vi "myPID.vi"(11 "Numeric":dbl format="%#_13g") -> (3 "Numeric 2":dbl)   [LabVIEW 2018]
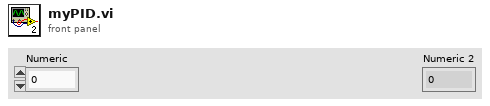
[diagram p1: front panel]
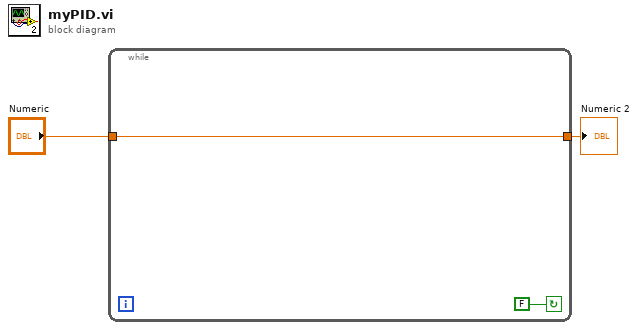
[diagram p0: block diagram]
diagram:
  n1 = while {
    tunnel: "Numeric" -> [w4]
    tunnel: [w4] -> w1
    stop <- FALSE continue-if-true
  }
  "Numeric 2" <- w1
